vi "sensorIDtest.vi"() -> ()   [LabVIEW 2021, in "Test VIs.lvclass"]
uses:
  Test VIs.lvclass
panel:
  out "Sensor ID Location":dbl[][](array[numeric])
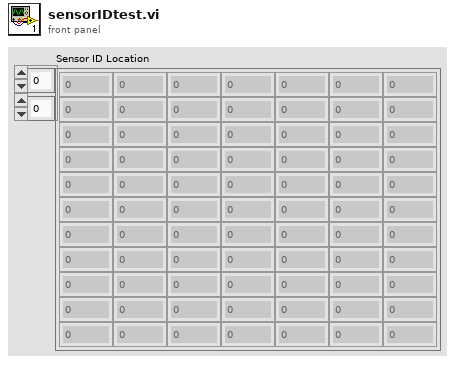
[diagram p1: front panel]
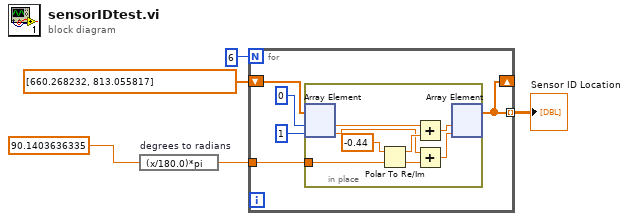
[diagram p0: block diagram]
diagram:
  n1 = expression code="(x/180.0)*pi" "degrees to radians"(90.1403636335 ("theta")) -> (w1:dbl)
  n2 = for {
    N: 6 -> [_]
    shift-right: [w6] -> _
    shift-left: dbl[] [660.268232, 813.055817] ("Sensor ID Location") -> [w8]
    tunnel: w1 -> [w7]
    tunnel: [w6] -> w3 mode=indexing
    n3 = in-place {
      in-place-border: w7 -> [w11]
      n4 = in-place-array #1(w8, 0, 1) -> (w15:dbl, w14:dbl)
      n5 = Polar To Re/Im(2:w11, 3:-0.44 ("r")) -> (0:w16:dbl, 1:w17:dbl)
      n6 = Add(x=w15, y=w17) -> (x+y=w12:dbl)
      n7 = Add(x=w14, y=w16) -> (x+y=w13:dbl)
      n8 = in-place-array #1(w12, w13) -> (w6:dbl[])  [unwired: 2 out]
    }
  }
  "Sensor ID Location" <- w3
